vi "InternalErrorOccured.vi"(4 "String":refnum<vi>, 5 "Event Data":cluster{"sender":refnum<k24>, "e":refnum<k24>}, 6 "Control Ref":refnum<k24>, 7 "Event Common Data":T1) -> ()   [LabVIEW 2018]
uses:
  C:/Users/fg/Documents/UniversalRobots.vi/LabVIEW_2024/UnderAutomation.UniversalRobots/lib/UnderAutomation.UniversalRobots.dll
  LabVIEW_2024/UnderAutomation.UniversalRobots/lib/UnderAutomation.UniversalRobots.dll
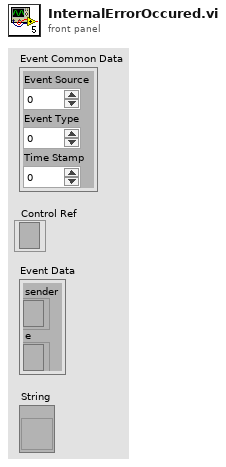
[diagram p1: front panel]
types:
  T1 = cluster{"Event Source":i32, "Event Type":u32, "Time Stamp":u32}
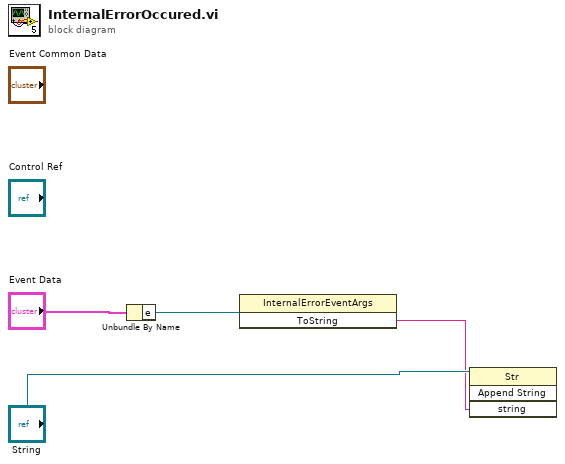
[diagram p0: block diagram]
diagram:
  n1 = Unbundle By Name("Event Data") -> ("e"=w3:refnum<k24>)
  n2 = invoke class="InternalErrorEventArgs" method="ToString"(reference=w3) -> ("ToString"=w1:string)  [unwired: 2 in, 2 out]
  n3 = invoke class="Str" method="Append String"(reference="String", "string"=w1) -> ()  [unwired: 2 in, 4 out]
